vi "Get Selection from NodeBrowserWF.vi"(8 "error in (no error)":errorcluster, 11 "NodeBrowserRefs":refnum<k24>[](array[refnum])) -> (0 "error out":errorcluster, 3 "Array":T1[](array[typedef]) {"Data Type" items=["Signed", "Unsigned", "IEEE Float"]})   [LabVIEW 2013, in "Protection and Rolling Counter Addon System Explorer.lvlib"]
uses:
  Protection and Rolling Counter Addon System Explorer.lvlib
  Shared/Types/InputChannelConfiguration.ctl
  NationalInstruments.VeriStand.SystemStorageUI
  NationalInstruments.VeriStand.SystemStorage
  Shared/Protection and Rolling Counter Addon Shared.lvlib
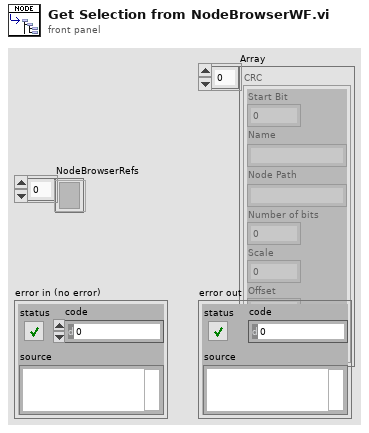
[diagram p1: front panel]
types:
  T1 = typedef "Protection and Rolling Counter Addon Shared.lvlib/InputChannelConfiguration.ctl" = cluster{"Start Bit":i32, "Name":string, "Node Path":string, "Number of bits":i32, "Scale":dbl, "Offset":dbl, "Data Type":u32}
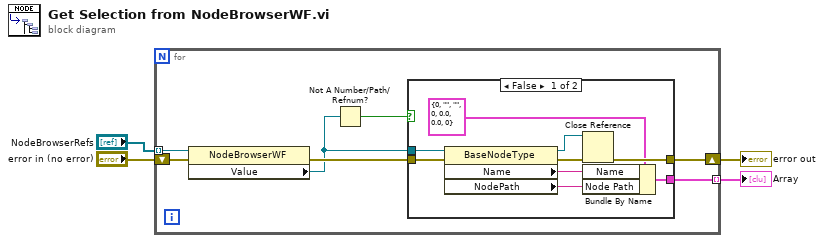
[diagram p0: block diagram]
diagram:
  n1 = for {
    shift-right: [w9] -> w3
    shift-left: "error in (no error)" -> [w11]
    tunnel: "NodeBrowserRefs" -> [w8] mode=indexing
    tunnel: [w7] -> w4 mode=indexing
    n2 = property class="NodeBrowserWF"(reference=w8, error in=w11) -> (error out=w10:errorcluster, "Value"=w6:refnum<k24>)  [unwired: 1 out]
    n3 = Not A Number/Path/Refnum?(number/path/refnum=w6) -> (NaN/Path/Refnum?=w5:bool)
    n4 = case shown="False" w5 {
      tunnel: w10 -> [w20 w21]
      tunnel: [w14 w21] -> w9
      tunnel: [w16 _] -> w7
      tunnel: w6 -> [w15 _]
      frame False {
        n5 = property class="BaseNodeType"(reference=w15, error in=w20) -> (reference out=w13:refnum<k24>, error out=w19:errorcluster, "Name"=w18:string, "NodePath"=w17:string)
        n6 = Close Reference(reference=w13, error in (no error)=w19) -> (error out=w14:errorcluster)
        n7 = Bundle By Name(cluster=T1 {"Start Bit"=0, "Name"="", "Node Path"="", "Number of bits"=0, "Scale"=0.0, "Offset"=0.0, "Data Type"=0} ("CRC"), "Name"=w18, "Node Path"=w17) -> (w16:T1)
      }
      frame True {
      }
    }
  }
  "Array" <- w4
  "error out" <- w3
